vi "Get Channel Name.vi"(8 "error in (no error)":errorcluster, 10 "Node Path":string, 11 "NIVS.System Definition Root in":refnum<k24>) -> (0 "error out":errorcluster, 2 "Name":string, 3 "NIVS.System Definition Root out":refnum<k24>)   [LabVIEW 2014]
uses:
  NationalInstruments.VeriStand.SystemStorage
  NationalInstruments.VeriStand
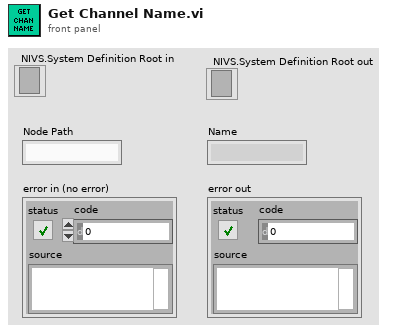
[diagram p1: front panel]
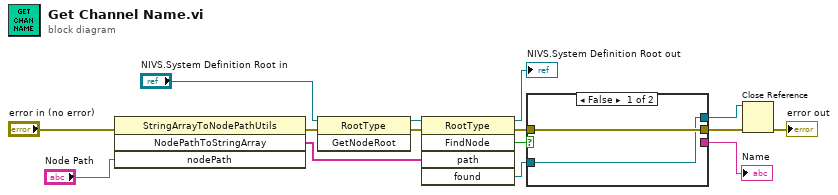
[diagram p0: block diagram]
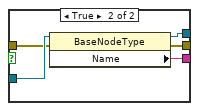
[diagram p2: hidden frame]
diagram:
  n1 = invoke class="StringArrayToNodePathUtils" method="NodePathToStringArray"(error in="error in (no error)", "nodePath"="Node Path") -> (error out=w10:errorcluster, "NodePathToStringArray"=w9:string[])  [unwired: 2 in, 2 out]
  n2 = invoke class="RootType" method="GetNodeRoot"(reference="NIVS.System Definition Root in", error in=w10) -> (reference out=w14:refnum<k24>, error out=w15:errorcluster)  [unwired: 1 in, 1 out]
  n3 = invoke class="RootType" method="FindNode"(reference=w14, error in=w15, "path"=w9) -> (reference out=→"NIVS.System Definition Root out":refnum<k24>, error out=w13:errorcluster, "FindNode"=w12:bool, "found"=w4:refnum<k24>)  [unwired: 2 in, 1 out]
  n4 = case shown="False" w12 {
    tunnel: w4 -> [w16 w22]
    tunnel: w13 -> [w17 w20]
    tunnel: [w17 w21] -> w11
    tunnel: [_ w19] -> w5
    tunnel: [w16 w18] -> w3
    frame False {
    }
    frame True {
      n5 = property class="BaseNodeType"(reference=w22, error in=w20) -> (reference out=w18:refnum<k24>, error out=w21:errorcluster, "Name"=w19:string)
    }
  }
  "Name" <- w5
  n6 = Close Reference(reference=w3, error in (no error)=w11) -> (error out=→"error out":errorcluster)
